vi "CamToGH_OffsetFinder.vi"() -> ()   [LabVIEW 2019]
panel:
  in  "Pos":enum16{"Left", "Right", "Top(Y+)", "Bot(Y-)"}(ring)
  in  "mm/pxel":dbl=0.0006823
  in  "NPxlY":dbl=2048.0
  in  "NPxlX":dbl=2448.0
  in  "Yoffset":dbl=117.072
  in  "Xoffset":dbl=30.285
  in  "FRightX":string="G1 X1234.6857703 Y1005.2548751 F100\rG1 Z64.0510003"
  in  "FLeftX":string="G1 X1048.1983480 Y1008.4914097 F100\rG1 Z64.1449993"
  in  "FidFinder":bool=TRUE
  in  "PickPlace":bool
  in  "GotoFidBot(Y-)":string="G1 X1141.9174162 Y912.2486534 F100\rG1 Z64.1745949"
  in  "GotoFidTop(Y+)":string="G1 X1137.9635488 Y1098.7360318 F100\rG1 Z64.1745939"
  out "NumCirclesFoundF1":i32
  out "Image":T1(plugin-control)
  out "CircleCenterGH(mm)":string
  out "CenterPosition":cluster{"X":sgl, "Y":sgl}
  out "Radius":dbl
  in  "DropToolAt":string="G1 X875.4470621\tY919.833414"
  in  "RotationGH":string="G1 U182.0"
  in  "PickPlateFrom":string="G1 X1173.241874\tY1124.027858"
  in  "PickToolFrom":string="G1 Z0\nG1 U2.0\nG1 X875.4470621\tY919.83341"
  in  "DropTool":i32=10
  in  "DropPlate":u32=42
  in  "PickPlate":u32=50
  in  "PickTool":u32=42
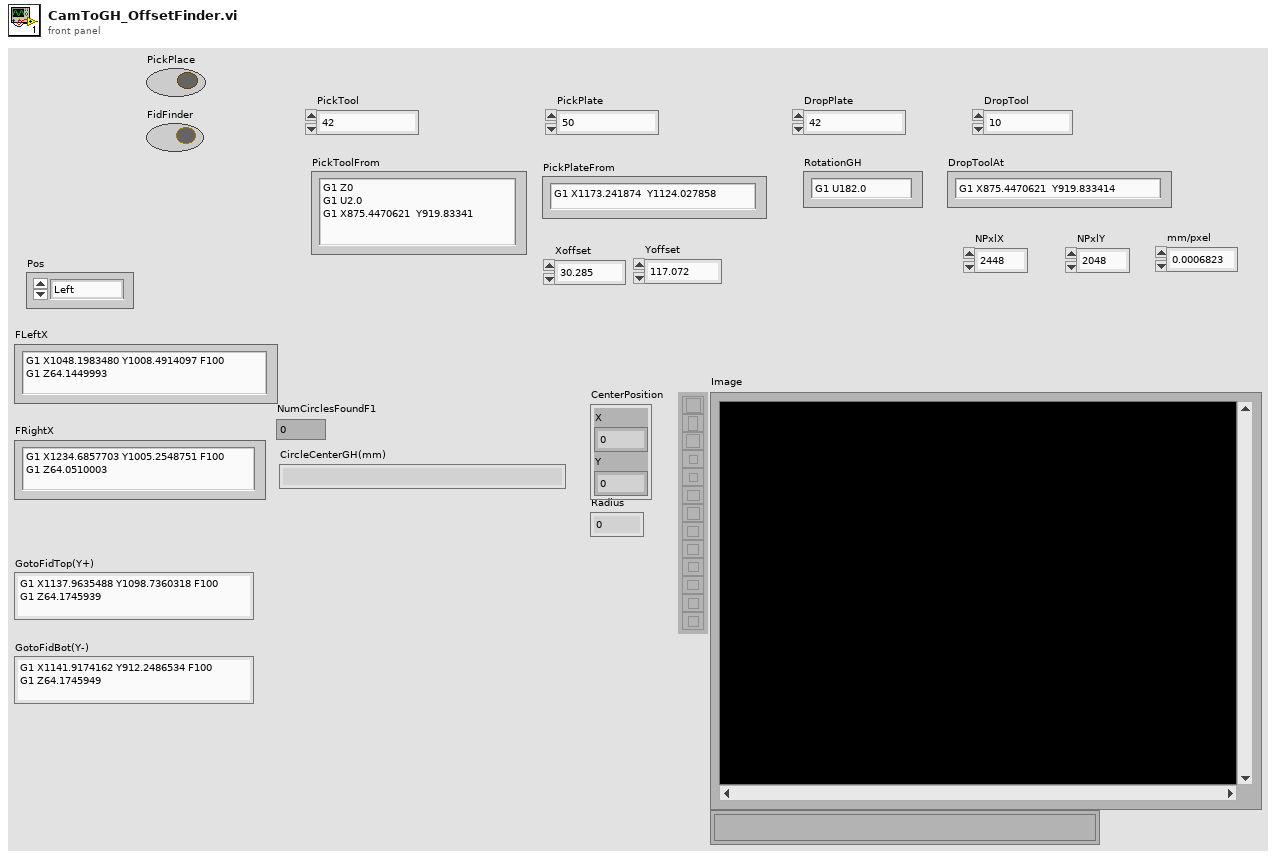
[diagram p1: front panel]
types:
  T1 = typedef "IMAQ Image.ctl" = refnum<image>
  T2 = cluster{"Position":cluster{"X":sgl, "Y":sgl}, "Radius":dbl, "Score":dbl}
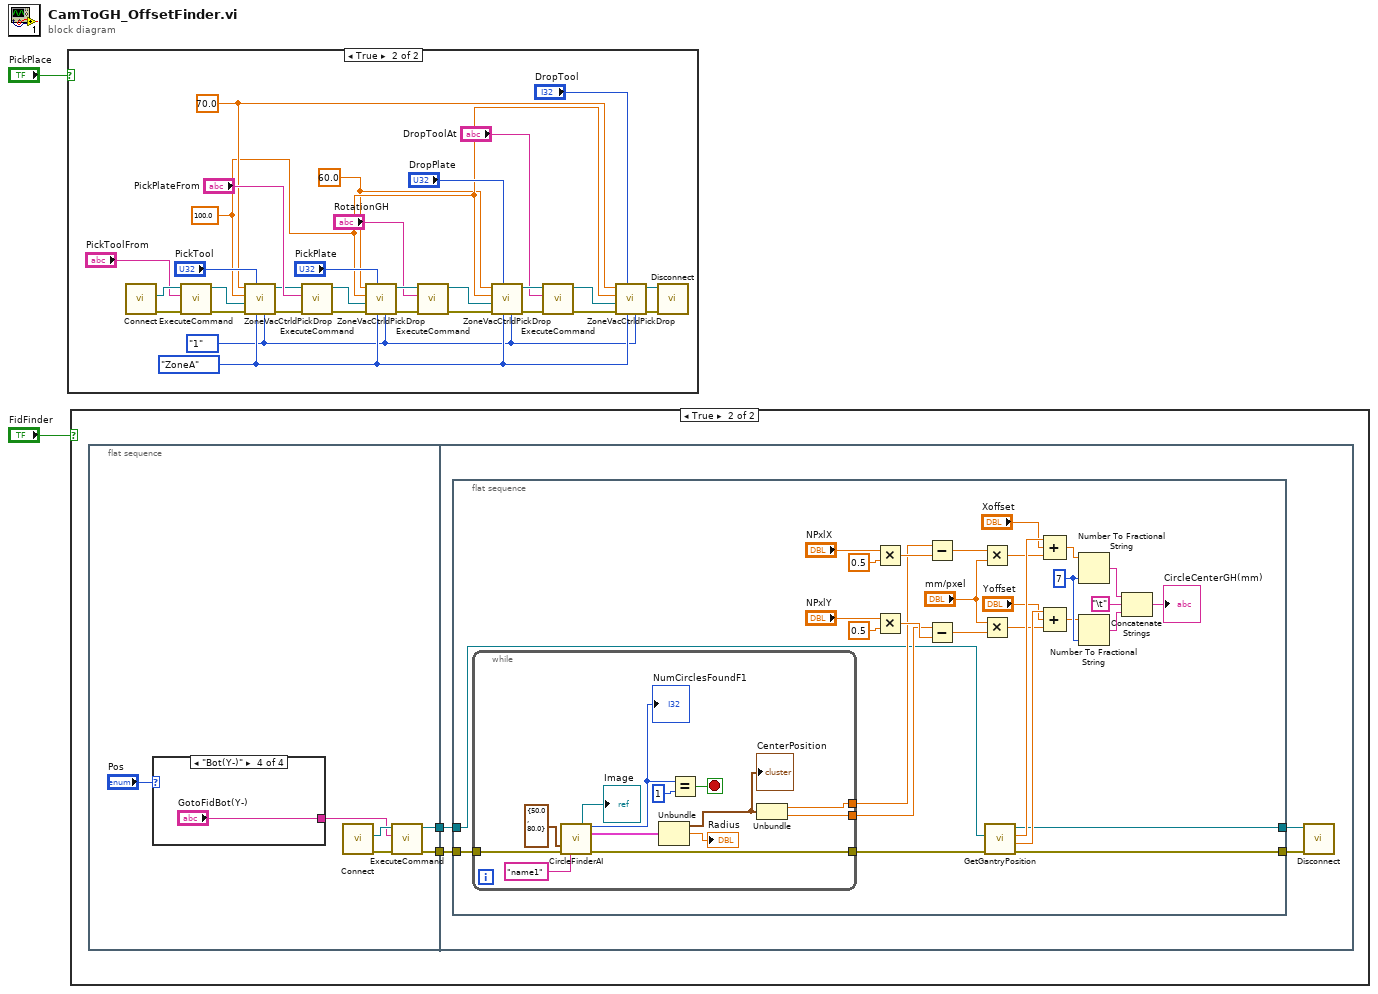
[diagram p0: block diagram]
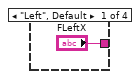
[diagram p3: hidden frame]
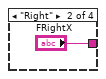
[diagram p4: hidden frame]
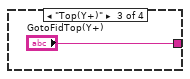
[diagram p5: hidden frame]
diagram:
  n1 = case shown="True" "PickPlace" {
    frame False {
    }
    frame True {
      w9 = 60.0 ("Z")
      w11 = 70.0 ("Z")
      w3 = enum16{"1", "2"}."1" ("Position")
      w4 = enum16{"ZoneA", "ZoneB", "ZoneC", "ZoneD"}."ZoneA" ("Zone")
      w10 = 100.0 ("Zspeed")
      n2 = call "Connect.vi"() -> ("error out"=w33:errorcluster, "controller"=w32:refnum<k24>)  [unwired: 10 in]
      n3 = call "ExecuteCommand.vi"("error in (no error)"=w33, "Command Code"="PickToolFrom", "controller in"=w32) -> ("error out"=w31:errorcluster, "controller out"=w30:refnum<k24>)  [unwired: 6 in, 1 out]
      n4 = call "ZoneVacCtrldPickDrop.vi"("Position"=w3, "Zone"=w4, "VacuumState"="PickTool", "error in (no error)"=w31, "controller in"=w30, "Zspeed"=w10, "Z"=w11) -> ("error out"=w25:errorcluster, "controller out"=w26:refnum<k24>)  [unwired: 3 in]
      n5 = call "ExecuteCommand.vi"("error in (no error)"=w25, "Command Code"="PickPlateFrom", "controller in"=w26) -> ("error out"=w23:errorcluster, "controller out"=w24:refnum<k24>)  [unwired: 6 in, 1 out]
      n6 = call "ZoneVacCtrldPickDrop.vi"("Position"=w3, "Zone"=w4, "VacuumState"="PickPlate", "error in (no error)"=w23, "controller in"=w24, "Zspeed"=w10, "Z"=w9) -> ("error out"=w19:errorcluster, "controller out"=w21:refnum<k24>)  [unwired: 3 in]
      n7 = call "ExecuteCommand.vi"("error in (no error)"=w19, "Command Code"="RotationGH", "controller in"=w21) -> ("error out"=w16:errorcluster, "controller out"=w18:refnum<k24>)  [unwired: 6 in, 1 out]
      n8 = call "ZoneVacCtrldPickDrop.vi"("Position"=w3, "Zone"=w4, "VacuumState"="DropPlate", "error in (no error)"=w16, "controller in"=w18, "Zspeed"=w10, "Z"=w9) -> ("error out"=w14:errorcluster, "controller out"=w15:refnum<k24>)  [unwired: 3 in]
      n9 = call "ExecuteCommand.vi"("error in (no error)"=w14, "Command Code"="DropToolAt", "controller in"=w15) -> ("error out"=w12:errorcluster, "controller out"=w8:refnum<k24>)  [unwired: 6 in, 1 out]
      n10 = call "ZoneVacCtrldPickDrop.vi"("Position"=w3, "Zone"=w4, "VacuumState"="DropTool", "error in (no error)"=w12, "controller in"=w8, "Zspeed"=w10, "Z"=w11) -> ("error out"=w6:errorcluster, "controller out"=w5:refnum<k24>)  [unwired: 3 in]
      n11 = call "Disconnect.vi"("error in (no error)"=w6, "controller"=w5) -> ()  [unwired: 9 in, 1 out]
    }
  }
  n12 = case shown="True" "FidFinder" {
    frame False {
    }
    frame True {
      n13 = flat-sequence {
        tunnel: [w39] -> w35
        tunnel: [w38] -> w34
        tunnel: w35 -> [w47]
        tunnel: w34 -> [w49]
        frame #0 {
          n14 = case shown="\"Bot(Y-)\"" "Pos" {
            tunnel: ["FLeftX" "FRightX" "GotoFidTop(Y+)" "GotoFidBot(Y-)"] -> w36
            frame "Left", Default {
            }
            frame "Right" {
            }
            frame "Top(Y+)" {
            }
            frame "Bot(Y-)" {
            }
          }
          n15 = call "Connect.vi"() -> ("error out"=w41:errorcluster, "controller"=w40:refnum<k24>)  [unwired: 10 in]
          n16 = call "ExecuteCommand.vi"("error in (no error)"=w41, "Command Code"=w36, "controller in"=w40) -> ("error out"=w39:errorcluster, "controller out"=w38:refnum<k24>)  [unwired: 6 in, 1 out]
        }
        frame #1 {
          n17 = flat-sequence {
            tunnel: w49 -> [w53]
            tunnel: [w52] -> w48
            tunnel: w47 -> [w51]
            tunnel: [w50] -> w46
            frame #0 {
              w78 = i16 7 ("precision (6)")
              n18 = while {
                tunnel: [w80] -> w54
                tunnel: [w90] -> w67
                tunnel: [w89] -> w66
                tunnel: w51 -> [w79]
                stop <- w86 stop-if-true
                n19 = call "CircleFinderAI.vi"("Circle Descriptor"=cluster{"Min Radius":dbl, "Max Radius":dbl} {"Min Radius"=50.0, "Max Radius"=80.0}, "error in (no error)"=w79, "Image Name"="name1") -> ("Image"=→"Image":T1, "NumCirclesFound"=w81:i32, "Circle0"=w82:T2, "error out"=w80:errorcluster)  [unwired: 8 in, 1 out]
                "NumCirclesFoundF1" <- w81
                n20 = Unbundle(w82) -> ("Position"=w91:cluster{"X":sgl, "Y":sgl}, "Radius"=→"Radius":dbl)  [unwired: 1 out]
                "CenterPosition" <- w91
                n21 = Equal?(x=w81, y=1) -> (x = y?=w86:bool)
                n22 = Unbundle(w91) -> ("X"=w90:sgl, "Y"=w89:sgl)
              }
              n23 = Multiply(x="NPxlX", y=0.5) -> (x*y=w72:dbl)
              n24 = Multiply(x="NPxlY", y=0.5) -> (x*y=w73:dbl)
              n25 = Subtract(x=w67, y=w72) -> (x-y=w65:dbl)
              n26 = Subtract(x=w66, y=w73) -> (x-y=w63:dbl)
              n27 = Multiply(x=w65, y="mm/pxel") -> (x*y=w60:dbl)
              n28 = Multiply(x="mm/pxel", y=w63) -> (x*y=w57:dbl)
              n29 = call "GetGantryPosition.vi"("error in (no error)"=w54, "Controller In"=w53) -> ("error out"=w50:errorcluster, "Position Y"=w59:dbl, "Position X"=w62:dbl, "controller out"=w52:refnum<k24>)  [unwired: 3 in, 3 out]
              n30 = Compound Arithmetic op=ADD(w62, "Xoffset", w60) -> (w56:dbl)
              n31 = Compound Arithmetic op=ADD(w59, "Yoffset", w57) -> (w55:dbl)
              n32 = Number To Fractional String(number=w56, precision (6)=w78) -> (F-format string=w77:string)  [unwired: 2 in]
              n33 = Number To Fractional String(number=w55, precision (6)=w78) -> (F-format string=w75:string)  [unwired: 2 in]
              n34 = Concatenate Strings(w77, "\t", w75) -> (→"CircleCenterGH(mm)":string)
            }
          }
          n35 = call "Disconnect.vi"("error in (no error)"=w46, "controller"=w48) -> ()  [unwired: 9 in, 1 out]
        }
      }
    }
  }
